vi "bytesplitter.vi"(11 "Byte":u8 format="%.0x") -> (2 "Low Nibble":u8, 3 "High Nibble":u8 format="%.0x")   [LabVIEW 2020, in "midi-file.lvclass"]
uses:
  midi-file.lvclass
  midi-file.lvclass/midi-file.ctl
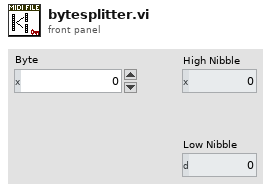
[diagram p1: front panel]
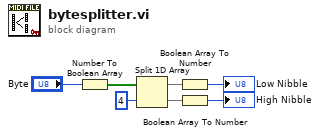
[diagram p0: block diagram]
diagram:
  n1 = Number To Boolean Array(number="Byte") -> (Boolean array=w6:bool[])
  n2 = Split 1D Array(array=w6, index=4) -> (first subarray=w5:bool[], second subarray=w4:bool[])
  n3 = Boolean Array To Number(Boolean array=w5) -> (number=→"Low Nibble":u8)
  n4 = Boolean Array To Number(Boolean array=w4) -> (number=→"High Nibble":u8)
